vi "Pot Lines.vi"(8 "error in":errorcluster, 10 "Potting Lines":T1[](array[typedef]), 11 "SyringeTool in":refnum<class "SyringeTool Class.lvclass">) -> (0 "error out":errorcluster, 3 "SyringeTool out":refnum<class "SyringeTool Class.lvclass">)   [LabVIEW 2011, in "SyringeTool Class.lvclass"]
uses:
  SyringeTool Class.lvclass
  Type Definitions/Potting Line.ctl
  Vec3d Class/Vec3d Class.lvclass
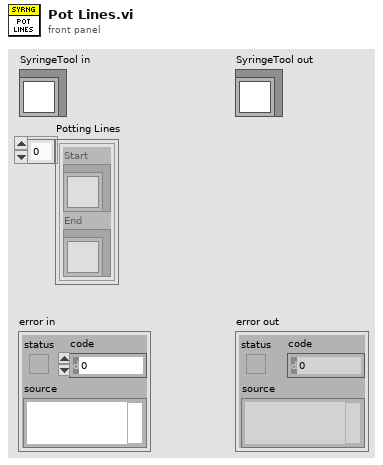
[diagram p1: front panel]
types:
  T1 = typedef "Potting Line.ctl" = cluster{"Start":refnum<class "Vec3d Class.lvclass">, "End":refnum<class "Vec3d Class.lvclass">}
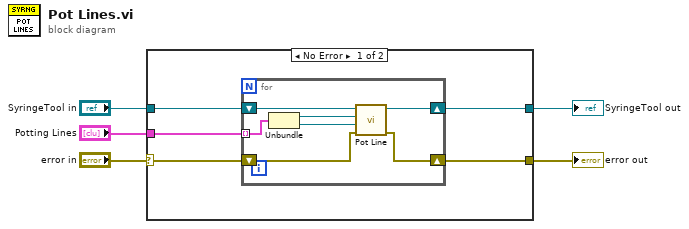
[diagram p0: block diagram]
diagram:
  n1 = case shown="No Error" "error in" {
    selector: "error in" -> [w8 w19]
    tunnel: [w6 w19] -> w4
    tunnel: [w7 w18] -> w2
    tunnel: "SyringeTool in" -> [w9 w18]
    tunnel: "Potting Lines" -> [w10 _]
    frame No Error {
      n2 = for {
        tunnel: w10 -> [w15] mode=indexing
        shift-right: [w12] -> w7
        shift-left: w9 -> [w17]
        shift-right: [w11] -> w6
        shift-left: w8 -> [w16]
        n3 = Unbundle(w15) -> ("Start"=w14:refnum<class "Vec3d Class.lvclass">, "End"=w13:refnum<class "Vec3d Class.lvclass">)
        n4 = call-dynamic "Pot Line.vi"("error in"=w16, "End Position"=w13, "Start Position"=w14, "SyringeTool in"=w17) -> ("error out"=w11:errorcluster, "SyringeTool out"=w12:refnum<class "SyringeTool Class.lvclass">)  [unwired: 6 in]
      }
    }
    frame Error {
    }
  }
  "error out" <- w4
  "SyringeTool out" <- w2
